vi "Hall.vi"() -> ()   [LabVIEW 2018]
uses:
  <vilib>/Utility/file.llb/Read Delimited Spreadsheet (DBL).vi
  <vilib>/Utility/file.llb/Write Delimited Spreadsheet (DBL).vi
panel:
  in  "Save output":bool
  in  "Flatness":dbl=0.05
  out "R Hall mean":dbl
  out "XY Graph 2":cluster{"Field":dbl[], dbl[]}[](graph)
  in  "Bin size":dbl=0.1
  out "XY Graph":cluster{dbl[], dbl[]}[](graph)
  in  "Signal channel":string="LakeShore 370 (20) R"
  in  "Field channel":string="IPS120 (25) Field"
  in  "Group":string="p"
  in  "File Path Control":path
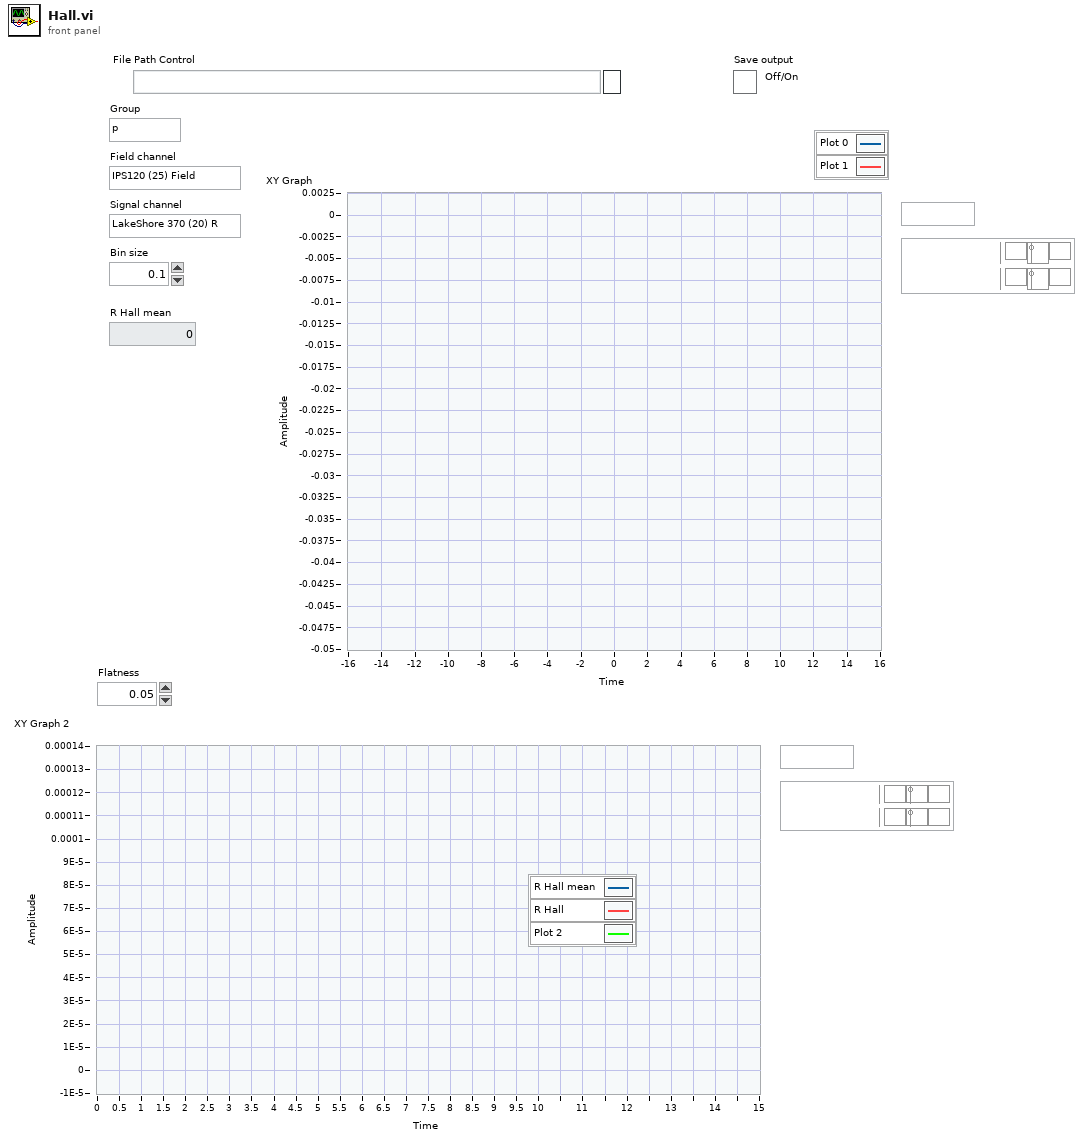
[diagram p1: front panel]
types:
  T1 = enum16{"open", "open or create", "create or replace", "create", "open (read-only)"}
  T2 = cluster{"Binned data":dbl[], "Binned data":dbl[]}
  T3 = cluster{"Binned data":dbl[], "Binned data":dbl[]}[]
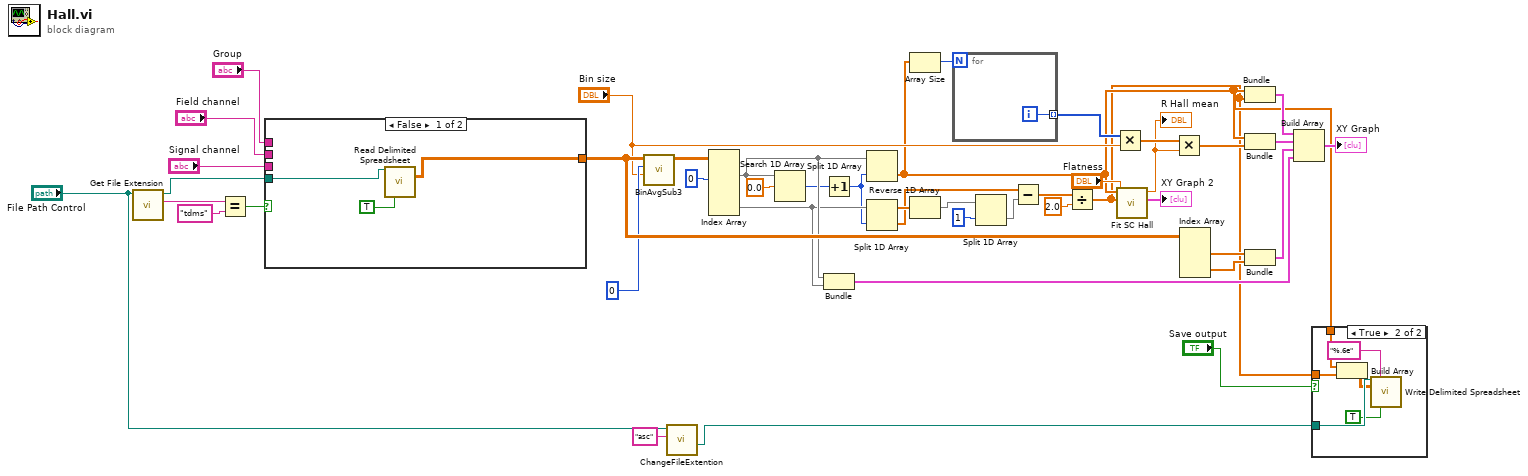
[diagram p0: block diagram]
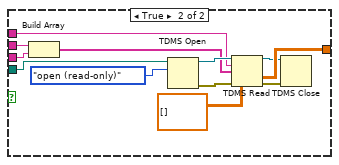
[diagram p3: hidden frame]
diagram:
  n1 = call <vilib>:"Get File Extension.vi"("file"="File Path Control") -> ("lowercase file extension"=w10:string, "dup file"=w11:path)  [unwired: 6 in, 3 out]
  n2 = Equal?(x=w10, y="tdms") -> (x = y?=w8:bool)
  n3 = case shown="False" w8 {
    tunnel: w11 -> [w47 w59]
    tunnel: "Group" -> [_ w55]
    tunnel: "Field channel" -> [_ w54]
    tunnel: "Signal channel" -> [_ w52]
    tunnel: [w46 w50] -> w38
    frame False {
      n4 = call-poly <vilib>:"Read Delimited Spreadsheet.vi"("file path (dialog if empty)"=w47, "transpose? (F)"=TRUE) -> ("all rows"=w46:dbl[][])  [unwired: 8 in, 5 out]
    }
    frame True {
      n5 = Build Array(w54, w52) -> (w53:string[])
      n6 = TDMS Open(10:T1."open (read-only)" ("operation (0:open)"), 11:w59) -> (0:w56:errorcluster, 3:w57:refnum<k34>)  [unwired: 5 in]
      n7 = TDMS Read(0:w57, 5:w55, 7:w53, 11:w56, 12:dbl[][] []) -> (4:w48:refnum<k34>, 10:w50:dbl[][], 15:w49:errorcluster)  [unwired: 3 in, 3 out]
      n8 = TDMS Close(8:w49, 11:w48) -> ()  [unwired: 2 out]
    }
  }
  n9 = call "BinAvgSub3.vi"("Bin size"="Bin size", "X coumn index"=0, "Data in"=w38) -> ("Binned data"=w35:dbl[][])  [unwired: 2 in, 6 out]
  n10 = call "ChangeFileExtention.vi"("New extension"="asc", "File Path"="File Path Control") -> ("Path with new extension"=w3:path)  [unwired: 4 in, 5 out]
  n11 = Index Array(array=w35, index (col) #1=0 ("disabled index (col)")) -> (element #1=w31:dbl[], element #3=w29:dbl[])  [unwired: 5 in, 1 out]
  n12 = Search 1D Array(1D array=w31, element=0.0) -> (index of element=w30:i32)  [unwired: 1 in]
  n13 = Increment(x=w30) -> (x+1=w28:i32)
  n14 = Bundle("Binned data"=w31, "Binned data"=w29) -> (w34:T2)  [unwired: 1 in]
  n15 = Split 1D Array(array=w31, index=w28) -> (second subarray=w2:dbl[])  [unwired: 1 out]
  n16 = Split 1D Array(array=w29, index=w28) -> (first subarray=w27:dbl[], second subarray=w24:dbl[])
  n17 = Array Size(array=w2) -> (size(s)=w22:i32)
  n18 = Reverse 1D Array(array=w27) -> (reversed array=w26:dbl[])
  n19 = for {
    N: w22 -> [_]
    tunnel: [w60] -> w21 mode=indexing
    i -> [w60]
  }
  n20 = Split 1D Array(array=w26, index=1) -> (second subarray=w23:dbl[])  [unwired: 1 out]
  n21 = Subtract(x=w24, y=w23) -> (x-y=w17:dbl[])
  n22 = Divide(x=w17, y=2.0) -> (x/y=w1:dbl[])
  n23 = Multiply(x=w21, y="Bin size") -> (x*y=w14:dbl[])
  n24 = call "Fit SC Hall.vi"("Flatness"="Flatness", "Hall signal"=w1, "Field"=w2) -> ("XY Graph"=→"XY Graph 2":cluster{"Field":dbl[], dbl[]}[], "Mean"=w12:dbl)  [unwired: 7 in]
  "R Hall mean" <- w12
  n25 = Multiply(x=w14, y=w12) -> (x*y=w18:dbl[])
  n26 = Index Array(array=w38) -> (element #1=w40:dbl[], element #2=w39:dbl[])  [unwired: 4 in]
  n27 = Bundle(w2, w1) -> (w20:cluster{dbl[], dbl[]})  [unwired: 1 in]
  n28 = Bundle(w2, w18) -> (w19:cluster{dbl[], dbl[]})  [unwired: 1 in]
  n29 = Bundle("all rows"=w40, "all rows"=w39) -> (w42:cluster{"all rows":dbl[], "all rows":dbl[]})  [unwired: 1 in]
  n30 = Build Array(w20, w19, w42, w34) -> (→"XY Graph":T3)
  n31 = case shown="True" "Save output" {
    tunnel: w3 -> [_ w66]
    tunnel: w2 -> [_ w65]
    tunnel: w1 -> [_ w64]
    frame False {
    }
    frame True {
      n32 = Build Array(w65, w64) -> (w63:dbl[][])
      n33 = call-poly <vilib>:"Write Delimited Spreadsheet.vi"("file path (dialog if empty)"=w66, "format (%.3f)"="%.6e", "2D data"=w63, "transpose? (no:F)"=TRUE) -> ()  [unwired: 10 in, 2 out]
    }
  }
